vi "RR.vi"() -> ()   [LabVIEW 2017]
uses:
  <vilib>/Motion/FlexMotion/CustomControls/CustomControls.llb/Axis # (8 axes).flx
  <vilib>/Motion/FlexMotion/CustomControls/CustomControls.llb/AxisOrVectorSpace To Configure.flx
  <vilib>/Motion/FlexMotion/FunctionsVIs/Trajectory.llb/Load Accel/Decel in RPS/sec.flx
  <vilib>/Motion/FlexMotion/FunctionsVIs/AxisResourceConfig.llb/Enable Axes (8 axes).flx
  <vilib>/Motion/FlexMotion/FunctionsVIs/StartStopMotion.llb/Start Motion (8 axes).flx
  <vilib>/Motion/FlexMotion/FunctionsVIs/StartStopMotion.llb/Stop Motion (8 axes).flx
  <vilib>/Analysis/NI_AALBase.lvlib
panel:
  out "Array":dbl[](array[numeric])
  in  "stop 2":bool
  in  "samples":i32=1500
  out "Present (s)":dbl
  out "Elapsed Time (s)":dbl
  out "Time has Elapsed":bool
  in  "stop":bool
  in  "Start Rod":bool
  in  "Rod amplitude":dbl=50.0
  in  "Rod mean":dbl=100.0
  in  "Change Parameters":bool
  out "disc":dbl
  out "Bottom disk":dbl(graph)
  out "rod":dbl
  out "Rod":dbl(graph)
  in  "rod 2":bool caption="rod"
  in  "Value (200) 2":dbl=10.0 format="%.2f"
  in  "Start disk":bool
  in  "disc 2":bool
  in  "Bottom disk  2":dbl=120.0
  in  "Value (200)":dbl=10.0 format="%.2f"
  in  "Axis/VS Map (Disabled)":T1={"1"=FALSE, "2"=FALSE, "3"=TRUE, "4"=TRUE, "5"=FALSE, "6"=FALSE, "7"=FALSE, "8"=FALSE}
  # "Enable"
  # "Disable"
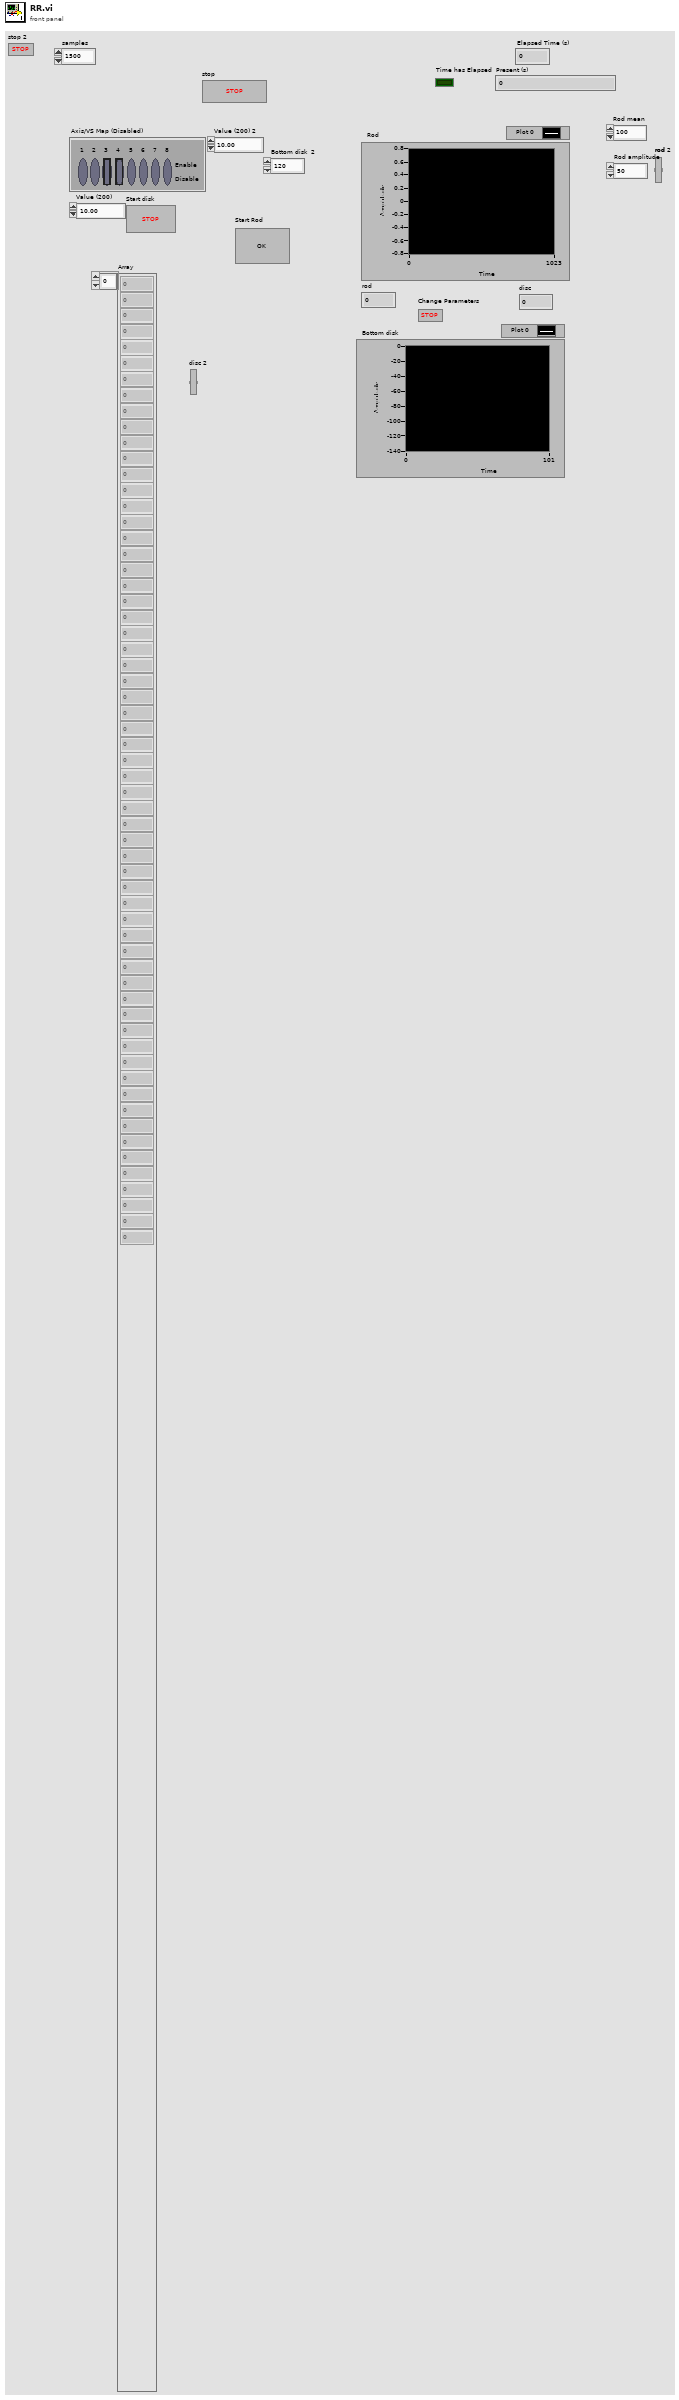
[diagram p1: front panel]
types:
  T1 = typedef "Axis # (8 axes).flx" = cluster{"1":bool, "2":bool, "3":bool, "4":bool, "5":bool, "6":bool, "7":bool, "8":bool}
  T2 = enum16{"Absolute Position", "Relative Position", "Velocity", "Relative to Cap Pos", "Modulus Position", "Absolute Contouring", "Relative Contouring"}
  T3 = typedef "Board Id" = u8
  T4 = typedef "AxisOrVectorSpace To Configure.flx" = u16
  T5 = typedef "Bd Id Out" = u8
  T6 = typedef "Resource Out (Enum).flx" = u16
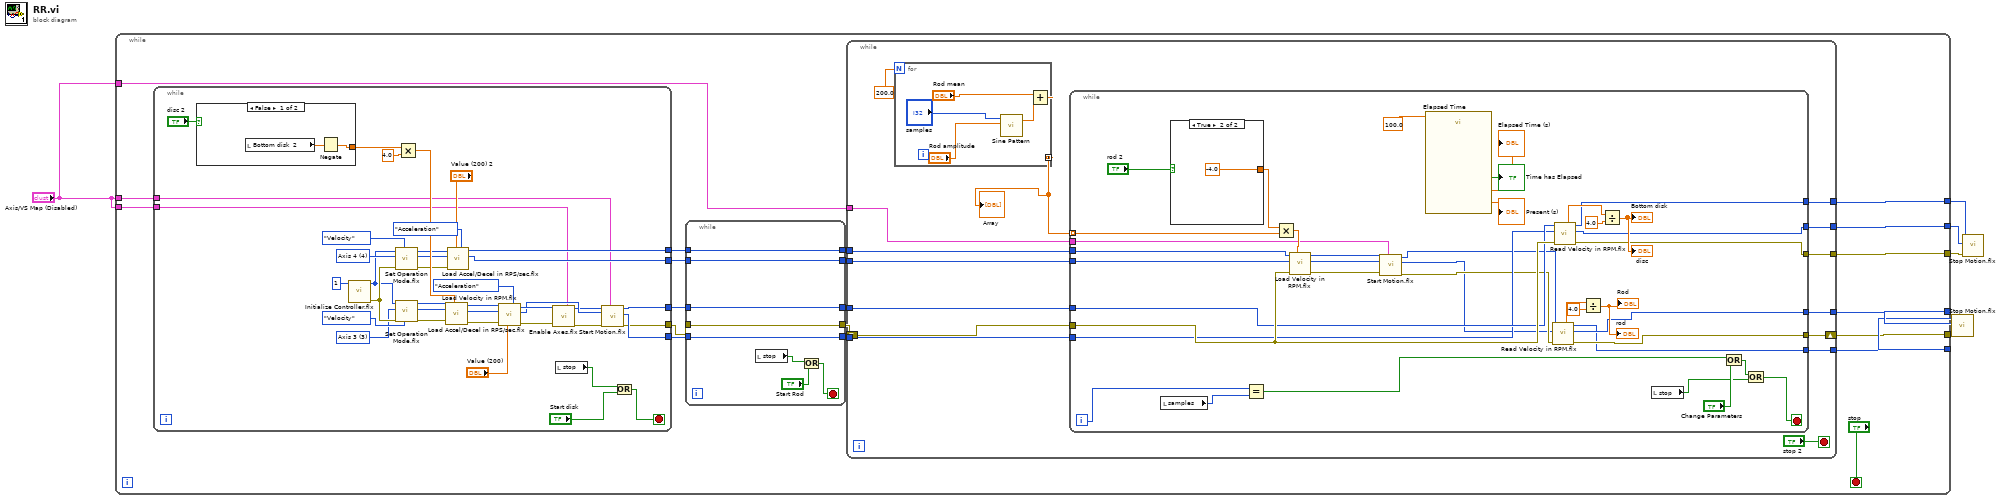
[diagram p0: block diagram]
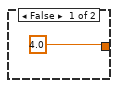
[diagram p2: hidden frame]
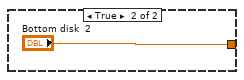
[diagram p3: hidden frame]
diagram:
  n1 = while {
    tunnel: [w22] -> w7
    tunnel: [w21] -> w6
    tunnel: [w20] -> w5
    tunnel: [w19] -> w4
    tunnel: [w18] -> w3
    tunnel: [w17] -> w2
    tunnel: "Axis/VS Map (Disabled)" -> [w15]
    tunnel: "Axis/VS Map (Disabled)" -> [w14]
    tunnel: "Axis/VS Map (Disabled)" -> [w13]
    stop <- "stop" stop-if-true
    n2 = while {
      tunnel: [w108] -> w23
      tunnel: [w107] -> w25
      tunnel: [w106] -> w24
      tunnel: [w103] -> w26
      tunnel: [w102] -> w27
      tunnel: w14 -> [w101]
      tunnel: w13 -> [w100]
      stop <- w97 stop-if-true
      w130 = T4 3 items=["Axis 1"=1, "Axis 2"=2, "Axis 3"=3, "Axis 4"=4, "Axis 5"=5, "Axis 6"=6, "Axis 7"=7, "Axis 8"=8, "Vector Space 1"=17, "Vector Space 2"=18, "Vector Space 3"=19, "Vector Space 4"=20] ("Axis or Vector Space")
      w134 = T4 4 items=["Axis 1"=1, "Axis 2"=2, "Axis 3"=3, "Axis 4"=4, "Axis 5"=5, "Axis 6"=6, "Axis 7"=7, "Axis 8"=8, "Vector Space 1"=17, "Vector Space 2"=18, "Vector Space 3"=19, "Vector Space 4"=20] ("Axis or Vector Space")
      n3 = case shown="False" "disc 2" {
        tunnel: [w137 "Bottom disk  2"] -> w115
        frame False {
          n4 = local read "Bottom disk  2"() -> (w136:dbl)
          n5 = Negate(x=w136) -> (-x=w137:dbl)
        }
        frame True {
        }
      }
      n6 = call <vilib>:"Initialize Controller.flx"("Board ID"=T3 1) -> ("error out"=w131:errorcluster, "Bd ID Out"=w129:T5)  [unwired: 7 in]
      n7 = call <vilib>:"Set Operation Mode.flx"("Position Mode (Absolute)"=T2."Velocity", "error in (no error)"=w131, "Axis or Vector Space"=w134, "Board ID"=w129) -> ("error out"=w112:errorcluster, "Resource Output"=w111:T6, "Bd ID Out"=w113:T5)  [unwired: 2 in]
      n8 = call <vilib>:"Set Operation Mode.flx"("Position Mode (Absolute)"=T2."Velocity", "error in (no error)"=w131, "Axis or Vector Space"=w130, "Board ID"=w129) -> ("error out"=w123:errorcluster, "Resource Output"=w127:T6, "Bd ID Out"=w128:T5)  [unwired: 2 in]
      n9 = Multiply(x=w115, y=4.0) -> (x*y=w114:dbl)
      n10 = call <vilib>:"Load Velocity in RPM.flx"("Velocity (500)"=w114, "error in (no error)"=w123, "Axis or Vector Space"=w127, "Board ID"=w128) -> ("error out"=w122:errorcluster, "Resource Output"=w125:T6, "Bd ID Out"=w126:T5)  [unwired: 3 in]
      n11 = call "Load Accel/Decel in RPS/sec.flx"("Selector (Both)"=enum16{"Both", "Acceleration", "Deceleration"}."Acceleration", "Value (200)"="Value (200) 2", "error in (no error)"=w112, "Axis or Vector Space"=w111, "Board ID"=w113) -> ("Resource Output"=w103:T6, "Bd ID Out"=w102:T5)  [unwired: 2 in, 1 out]
      n12 = call "Load Accel/Decel in RPS/sec.flx"("Selector (Both)"=enum16{"Both", "Acceleration", "Deceleration"}."Acceleration", "Value (200)"="Value (200)", "error in (no error)"=w122, "Axis or Vector Space"=w125, "Board ID"=w126) -> ("error out"=w121:errorcluster, "Resource Output"=w105:T6, "Bd ID Out"=w124:T5)  [unwired: 2 in]
      n13 = call-poly <vilib>:"Enable Axes.flx"("Axis Bitmap (Disabled)"=w100, "error in (no error)"=w121, "Board ID"=w124) -> ("error out"=w120:errorcluster, "Bd ID Out"=w104:T5)  [unwired: 5 in]
      n14 = local read "stop"() -> (w99:bool)
      n15 = call-poly <vilib>:"Start Motion.flx"("Axis/VS Map (Disabled)"=w101, "error in (no error)"=w120, "Axis or Vector Space"=w105, "Board ID"=w104) -> ("error out"=w106:errorcluster, "Resource Output"=w108:T6, "Bd ID Out"=w107:T5)  [unwired: 2 in]
      n16 = Or(x=w99, y="Start disk") -> (x .or. y?=w97:bool)
    }
    n17 = while {
      tunnel: w27 -> [w96]
      tunnel: [w96] -> w12
      tunnel: w26 -> [w95]
      tunnel: [w95] -> w11
      tunnel: w25 -> [w94]
      tunnel: [w94] -> w10
      tunnel: w24 -> [w93]
      tunnel: [w93] -> w9
      tunnel: w23 -> [w92]
      tunnel: [w92] -> w8
      stop <- w89 stop-if-true
      n18 = local read "stop"() -> (w91:bool)
      n19 = Or(x=w91, y="Start Rod") -> (x .or. y?=w89:bool)
    }
    n20 = while {
      tunnel: [w41] -> w21
      tunnel: [w40] -> w20
      tunnel: [w39] -> w19
      tunnel: [w38] -> w18
      tunnel: [w37] -> w17
      tunnel: w15 -> [w36]
      tunnel: w12 -> [w35]
      tunnel: w11 -> [w34]
      tunnel: w10 -> [w33]
      tunnel: w8 -> [w31]
      shift-right: [w42] -> w22
      shift-left: w9 -> [w32]
      stop <- "stop 2" stop-if-true
      n21 = for {
        N: 200.0 -> [_]
        tunnel: [w43] -> w28 mode=concatenating
        n22 = call <vilib>:"Sine Pattern.vi"("amplitude"="Rod amplitude", "samples"="samples") -> ("Sinusoidal Pattern"=w45:dbl[])  [unwired: 2 in, 1 out]
        n23 = Add(x="Rod mean", y=w45) -> (x+y=w43:dbl[])
      }
      "Array" <- w28
      n24 = while {
        tunnel: w28 -> [w84] mode=indexing
        tunnel: w36 -> [w82]
        tunnel: w31 -> [w72]
        tunnel: w33 -> [w73]
        tunnel: w32 -> [w74]
        tunnel: w34 -> [w71]
        tunnel: w35 -> [w67]
        tunnel: [w66] -> w42
        tunnel: [w65] -> w41
        tunnel: [w64] -> w40
        tunnel: [w63] -> w39
        tunnel: [w62] -> w38
        tunnel: [w61] -> w37
        i -> [w53]
        stop <- w58 stop-if-true
        n25 = local read "samples"() -> (w51:i32)
        n26 = case shown="True" "rod 2" {
          tunnel: [4.0 -4.0 ("y")] -> w85
          frame False {
          }
          frame True {
          }
        }
        n27 = Equal?(x=w53, y=w51) -> (x = y?=w52:bool)
        n28 = Multiply(x=w85, y=w84) -> (x*y=w83:dbl)
        n29 = call <vilib>:"Load Velocity in RPM.flx"("Velocity (500)"=w83, "error in (no error)"=w74, "Axis or Vector Space"=w71, "Board ID"=w67) -> ("error out"=w48:errorcluster, "Resource Output"=w49:T6, "Bd ID Out"=w50:T5)  [unwired: 3 in]
        n30 = call-poly <vilib>:"Start Motion.flx"("Axis/VS Map (Disabled)"=w82, "error in (no error)"=w48, "Axis or Vector Space"=w49, "Board ID"=w50) -> ("error out"=w70:errorcluster, "Resource Output"=w69:T6, "Bd ID Out"=w68:T5)  [unwired: 2 in]
        n31 = call "Elapsed Time"("Time Target (s)"=100.0) -> ("Present (s)"=→"Present (s)":dbl, "Elapsed Time (s)"=→"Elapsed Time (s)":dbl, "Time has Elapsed"=→"Time has Elapsed":bool)  [unwired: 11 in, 5 out]
        n32 = call <vilib>:"Read Velocity in RPM.flx"("error in (no error)"=w70, "Axis or Vector Space"=w69, "Board ID"=w68) -> ("error out"=w66:errorcluster, "Resource Output"=w65:T6, "Bd ID Out"=w64:T5, "Filtered Velocity"=w81:dbl)  [unwired: 3 in]
        n33 = call <vilib>:"Read Velocity in RPM.flx"("error in (no error)"=w74, "Axis or Vector Space"=w72, "Board ID"=w73) -> ("error out"=w63:errorcluster, "Resource Output"=w62:T6, "Bd ID Out"=w61:T5, "Filtered Velocity"=w76:dbl)  [unwired: 3 in]
        n34 = Divide(x=w81, y=4.0) -> (x/y=→"Rod" →"rod":dbl)
        n35 = Divide(x=w76, y=4.0) -> (x/y=→"Bottom disk" →"disc":dbl)
        n36 = local read "stop"() -> (w60:bool)
        n37 = Or(x=w52, y="Change Parameters") -> (x .or. y?=w59:bool)
        n38 = Or(x=w59, y=w60) -> (x .or. y?=w58:bool)
      }
    }
  }
  n39 = call-poly <vilib>:"Stop Motion.flx"("error in (no error)"=w7, "Axis or Vector Space"=w6, "Board ID"=w5) -> ()  [unwired: 4 in, 3 out]
  n40 = call-poly <vilib>:"Stop Motion.flx"("error in (no error)"=w4, "Axis or Vector Space"=w3, "Board ID"=w2) -> ()  [unwired: 4 in, 3 out]
